vi "Variant to Array.vi"(8 "error in (no error)":errorcluster, 11 "value":variant) -> (0 "error out":errorcluster, 3 "Array":dbl[](array[numeric]))   [LabVIEW 2016, in "LV to ITX.lvclass"]
uses:
  LV to ITX.lvclass
  <vilib>/Utility/error.llb/Error Cluster From Error Code.vi
  <vilib>/ErrorRing/Error Ring.xnode
  <vilib>/Utility/Data Type/NI_Data Type.lvlib
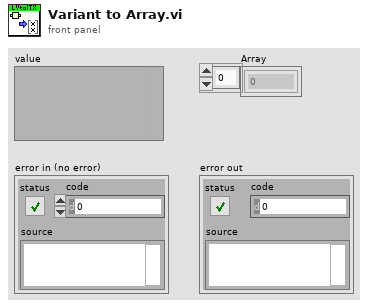
[diagram p1: front panel]
types:
  T1 = typedef "NI_Data Type.lvlib/Data Type.ctl" = enum8{"Invalid Type", "Void", "I8", "I16", "I32", "I64", "U8", "U16", "U32", "U64", "Single Float", "Double Float", "Extended Float", "Single Complex", "Double Complex", "Extended Complex", "Enum U8", "Enum U16", "Enum U32", "Enum U64", "Single Float With Unit", "Double Float With Unit", "Extended Float With Unit", "Single Complex with Unit", "Double Complex with Unit", "Extended Complex with Unit", "Boolean", "String", "Path", "Picture", "Tag", "Array", "Cluster", "Variant", "LV Variant", "Waveform", "Timestamp", "Digital Waveform", "Digital Data", "ExpressData", "Refnum", "External Data", "VI", "Poly VI", "LabVIEW Class Instance", "Fixed Point"}
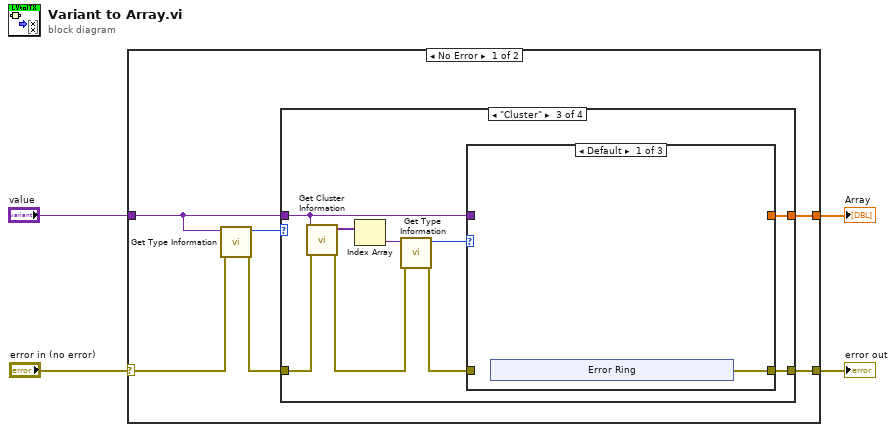
[diagram p0: block diagram]
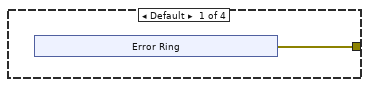
[diagram p2: hidden frame]
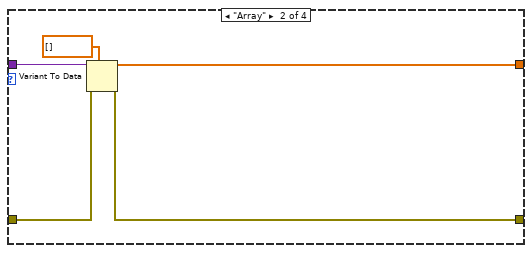
[diagram p3: hidden frame]
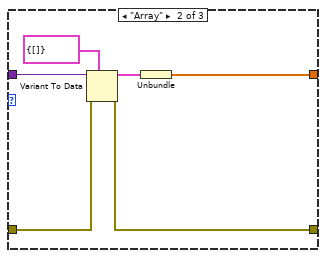
[diagram p4: hidden frame]
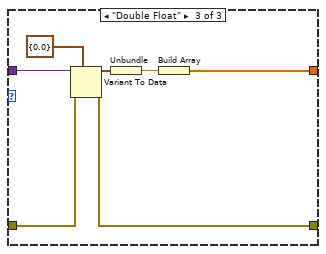
[diagram p5: hidden frame]
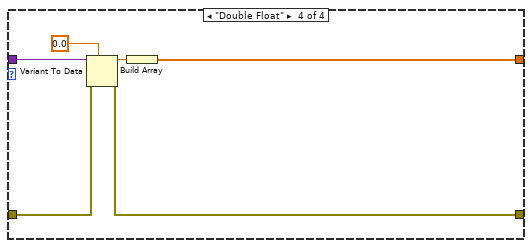
[diagram p6: hidden frame]
diagram:
  n1 = case shown="No Error" "error in (no error)" {
    selector: "error in (no error)" -> [w5 w54]
    tunnel: [w9 _] -> w4
    tunnel: [w6 w54] -> w3
    tunnel: "value" -> [w8 _]
    frame No Error {
      n2 = call <vilib>:"Get Type Information.vi"("error in (no error)"=w5, "Variant"=w8) -> ("error out"=w7:errorcluster, "Type"=w10:T1)  [unwired: 5 in, 3 out]
      n3 = case shown="\"Cluster\"" w10 {
        tunnel: [w11 w16 w24 w48] -> w6
        tunnel: [_ w19 w21 w50] -> w9
        tunnel: w8 -> [_ w18 w22 w52]
        tunnel: w7 -> [_ w17 w29 w49]
        frame Default {
          n4 = xnode "Error Ring"() -> ("error out"=w11:errorcluster)
        }
        frame "Array" {
          n5 = Variant To Data(error in=w17, type=dbl[] [], Variant=w18) -> (data=w19:dbl[], error out=w16:errorcluster)
        }
        frame "Cluster" {
          n6 = call <vilib>:"Get Cluster Information.vi"("error in (no error)"=w29, "Variant"=w22) -> ("error out"=w26:errorcluster, "Cluster Elements"=w28:variant[])  [unwired: 8 in]
          n7 = Index Array(array=w28) -> (element=w27:variant)  [unwired: 1 in]
          n8 = call <vilib>:"Get Type Information.vi"("error in (no error)"=w26, "Variant"=w27) -> ("error out"=w25:errorcluster, "Type"=w23:T1)  [unwired: 5 in, 3 out]
          n9 = case shown="Default" w23 {
            tunnel: [w30 w38 w44] -> w24
            tunnel: [_ w36 w46] -> w21
            tunnel: w25 -> [_ w39 w45]
            tunnel: w22 -> [_ w35 w41]
            frame Default {
              n10 = xnode "Error Ring"() -> ("error out"=w30:errorcluster)
            }
            frame "Array" {
              n11 = Variant To Data(error in=w39, type=cluster{dbl[]} {[]}, Variant=w35) -> (data=w40:cluster{dbl[]}, error out=w38:errorcluster)
              n12 = Unbundle(w40) -> (w36:dbl[])
            }
            frame "Double Float" {
              n13 = Variant To Data(error in=w45, type=cluster{dbl} {0.0}, Variant=w41) -> (data=w47:cluster{dbl}, error out=w44:errorcluster)
              n14 = Unbundle(w47) -> (w42:dbl)
              n15 = Build Array(w42) -> (w46:dbl[])
            }
          }
        }
        frame "Double Float" {
          n16 = Variant To Data(error in=w49, type=0.0, Variant=w52) -> (data=w53:dbl, error out=w48:errorcluster)
          n17 = Build Array(w53) -> (w50:dbl[])
        }
      }
    }
    frame Error {
    }
  }
  "Array" <- w4
  "error out" <- w3
